vi "Open Ref from Path.vi"(8 "error in (no error)":errorcluster, 11 "VI Reference Control in":refnum<class "Reference Control.lvclass">) -> (0 "error out":errorcluster, 3 "VI Reference Control out":refnum<class "Reference Control.lvclass">)   [LabVIEW 2016, in "Reference Control.lvclass"]
uses:
  Reference Control.lvclass
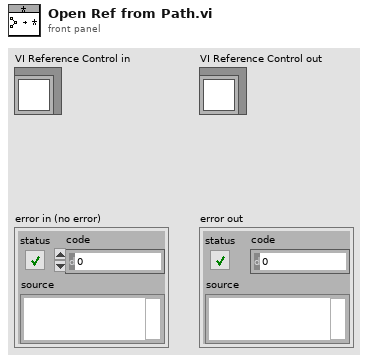
[diagram p1: front panel]
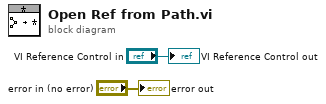
[diagram p0: block diagram]
diagram:
  "error out" <- "error in (no error)"
  "VI Reference Control out" <- "VI Reference Control in"
